vi "Execute EMS.vi"(8 "error in":errorcluster, 11 "Master Controller in":refnum<class "EMS User Interface.lvclass">) -> (0 "error out":errorcluster, 3 "Master Controller out":refnum<class "EMS User Interface.lvclass">)   [LabVIEW 2018, in "EMS User Interface Actor.lvlib" / "EMS User Interface.lvclass"]
uses:
  EMS User Interface.lvclass
  EMS User Interface.lvclass/EMS User Interface.ctl
  <vilib>/ActorFramework/Message Enqueuer/Message Enqueuer.lvclass/Message Enqueuer.ctl
  <vilib>/ActorFramework/Message Enqueuer/Enqueue.vi
  EMS Core/EMS Messages/Activate Init Msg/Activate Init Msg.lvclass
  C:/Program Files (x86)/National Instruments/LabVIEW 2018/vi.lib/ActorFramework/Message/Message.lvclass
  EMS Core/EMS Messages/Blackstart Init Msg/Blackstart Init Msg.lvclass
  EMS Core/EMS Messages/Shutdown Init Msg/Shutdown Init Msg.lvclass
  <vilib>/ActorFramework/Message Priority Queue/Priority Enqueue.vi
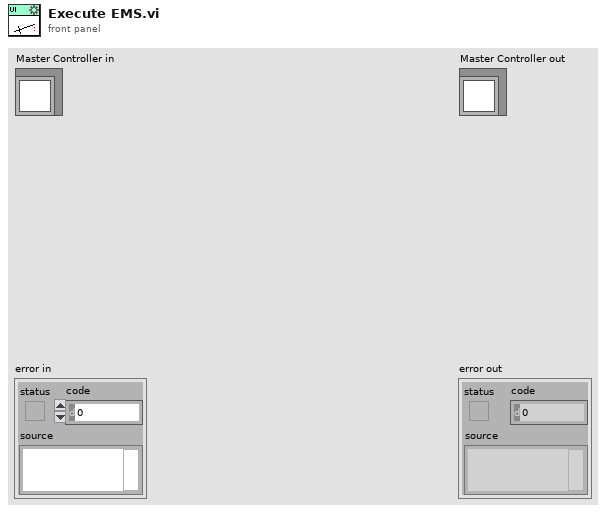
[diagram p1: front panel]
types:
  T1 = typedef "EMS Core.lvlib/EMS.lvclass/Microgrid State.ctl" = enum16{"Discovery", "Commissioning", "Activation", "Blackstart", "OnGrid", "OffGrid", "Island", "Resynchronization", "Manual", "Shutdown", "Stop"}
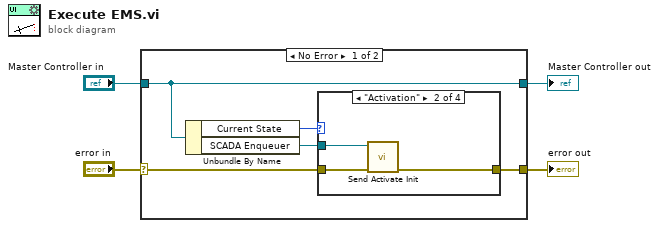
[diagram p0: block diagram]
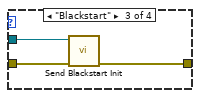
[diagram p3: hidden frame]
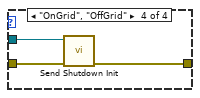
[diagram p4: hidden frame]
diagram:
  n1 = case shown="No Error" "error in" {
    selector: "error in" -> [w6 w21]
    tunnel: [w5 w21] -> w3
    tunnel: [w9 w20] -> w1
    tunnel: "Master Controller in" -> [w9 w20]
    frame No Error {
      n2 = Unbundle By Name(w9) -> ("Current State"=w8:T1, "SCADA Enqueuer"=w7:refnum<class "Message Enqueuer.lvclass">)
      n3 = case shown="\"Activation\"" w8 {
        tunnel: w7 -> [_ w13 w14 w17]
        tunnel: [w10 w12 w16 w18] -> w5
        tunnel: w6 -> [w10 w11 w15 w19]
        frame "Discovery", Default {
        }
        frame "Activation" {
          n4 = call "Send Activate Init.vi"("error in (no error)"=w11, "Message Enqueuer"=w13) -> ("error out"=w12:errorcluster)  [unwired: 8 in, 1 out]
        }
        frame "Blackstart" {
          n5 = call "Send Blackstart Init.vi"("error in"=w15, "Message Enqueuer"=w14) -> ("error out"=w16:errorcluster)  [unwired: 8 in, 1 out]
        }
        frame "OnGrid", "OffGrid" {
          n6 = call "Send Shutdown Init.vi"("error in (no error)"=w19, "Message Enqueuer"=w17) -> ("error out"=w18:errorcluster)  [unwired: 8 in, 1 out]
        }
      }
    }
    frame Error {
    }
  }
  "error out" <- w3
  "Master Controller out" <- w1
